vi "Remove Duplicate NCoincs.vi"(11 "Secondary hits sorted":T2(array[cluster])) -> (3 "Combined":T1(array[cluster]))   [LabVIEW 2016]
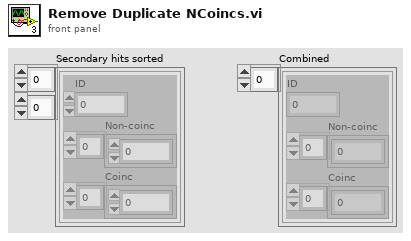
[diagram p1: front panel]
types:
  T1 = cluster{"ID":i8, "Non-coinc":u64[], "Coinc":u64[]}[]
  T2 = cluster{"ID":i8, "Non-coinc":u64[], "Coinc":u64[]}[][]
  T3 = cluster{"ID":i8, "Non-coinc":u64[], "Coinc":u64[]}
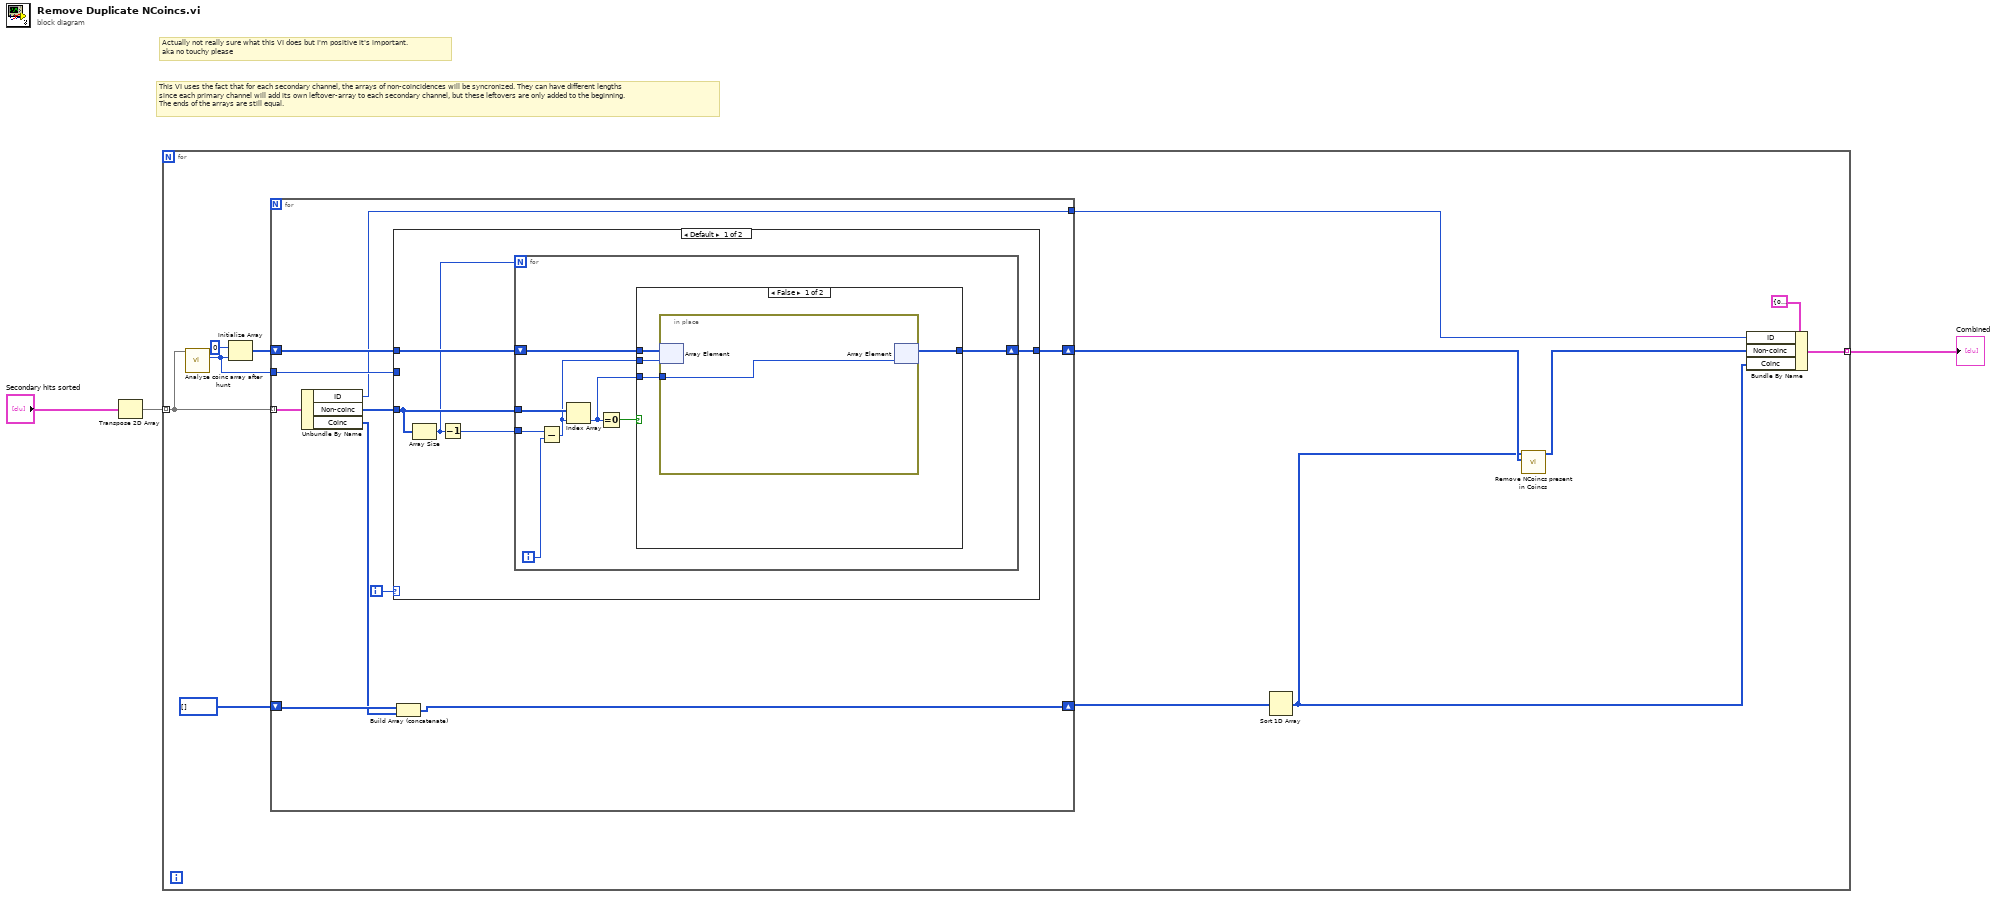
[diagram p0: block diagram]
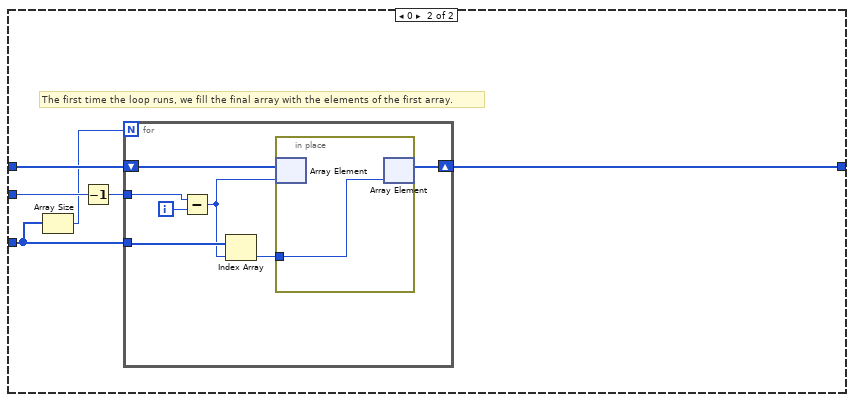
[diagram p3: hidden frame]
diagram:
  # "Actually not really sure what this VI does but I'm positive it's important.\naka no touchy please"
  # "This VI uses the fact that for each secondary channel, the arrays of non-coincidences will be syncronized. They can have different lengths\nsince each primary channel will add its own leftover-array to each secondary channel, but these leftovers are only added to the beginning.\nThe ends of the arrays are still equal."
  n1 = Transpose 2D Array(2D array="Secondary hits sorted") -> (transposed array=w2:T2)
  n2 = for {
    tunnel: w2 -> [w15] mode=indexing
    tunnel: [w7] -> w1 mode=indexing
    n3 = call "Analyze coinc array after hunt.vi"("Array"=w15) -> ("Largest array size"=w12:i32)  [unwired: 9 in, 1 out]
    n4 = Initialize Array(u64 0, w12) -> (w13:u64[])
    n5 = for {
      tunnel: w15 -> [w22] mode=indexing
      shift-right: [w18] -> w6
      shift-left: w13 -> [w25]
      tunnel: w12 -> [w23]
      shift-right: [w17] -> w9
      shift-left: u64[] [] ("initialized array") -> [w20]
      tunnel: [w16] -> w8
      i -> [w21]
      n6 = Unbundle By Name(w22) -> ("ID"=w16:i8, "Non-coinc"=w24:u64[], "Coinc"=w19:u64[])
      n7 = case shown="Default" w21 {
        tunnel: w25 -> [w28 w50]
        tunnel: w24 -> [w30 w45]
        tunnel: w23 -> [_ w48]
        tunnel: [w27 w47] -> w18
        frame Default {
          n8 = Array Size(array=w30) -> (size(s)=w26:i32)
          n9 = Decrement(x=w26) -> (x-1=w29:i32)
          n10 = for {
            N: w26 -> [_]
            tunnel: w30 -> [w38]
            tunnel: w29 -> [w37]
            shift-right: [w31] -> w27
            shift-left: w28 -> [w34]
            i -> [w36]
            n11 = Subtract(x=w37, y=w36) -> (x-y=w33:i32)
            n12 = Index Array(array=w38, index=w33) -> (element=w32:u64)
            n13 = Equal To 0?(x=w32) -> (x = 0?=w35:bool)
            n14 = case shown="False" w35 {
              tunnel: w34 -> [w42 w44]
              tunnel: w33 -> [w41 _]
              tunnel: w32 -> [w40 _]
              tunnel: [w39 w44] -> w31
              frame False {
                n15 = in-place {
                  in-place-border: w40 -> [w43]
                  n16 = in-place-array #1(w42, w41) -> ()  [unwired: 1 out]
                  n17 = in-place-array #1(w43) -> (w39:u64[])  [unwired: 1 out]
                }
              }
              frame True {
              }
            }
          }
        }
        frame 0 {
          # "The first time the loop runs, we fill the final array with the elements of the first array."
          n18 = Array Size(array=w45) -> (size(s)=w46:i32)
          n19 = Decrement(x=w48) -> (x-1=w49:i32)
          n20 = for {
            N: w46 -> [_]
            tunnel: w49 -> [w55]
            shift-right: [w54] -> w47
            shift-left: w50 -> [w57]
            tunnel: w45 -> [w53]
            i -> [w56]
            n21 = Subtract(x=w55, y=w56) -> (x-y=w51:i32)
            n22 = Index Array(array=w53, index=w51) -> (element=w52:u64)
            n23 = in-place {
              in-place-border: w52 -> [w58]
              n24 = in-place-array #2(w57, w51) -> ()  [unwired: 1 out]
              n25 = in-place-array #2(w58) -> (w54:u64[])  [unwired: 1 out]
            }
          }
        }
      }
      n26 = Build Array (concatenate)(w20, w19) -> (w17:u64[])
    }
    n27 = Sort 1D Array(array=w9) -> (sorted array=w5:u64[])
    n28 = call "Remove NCoincs present in Coincs.vi"("NCoincs"=w6, "Coincs"=w5) -> ("NCoincs cleaned"=w4:u64[])  [unwired: 9 in]
    n29 = Bundle By Name(cluster=T3 {"ID"=0, "Non-coinc"=[], "Coinc"=[]}, "ID"=w8, "Non-coinc"=w4, "Coinc"=w5) -> (w7:T3)
  }
  "Combined" <- w1
